vi "_Set Title.vi"(8 "error in (no error)":errorcluster, 9 "Title":string, 10 "Index":i32, 11 "Item_Refnums_Array":T1[](array[typedef])) -> (0 "error out":errorcluster, 3 "Item_Refnums_Array Out":T1[](array[typedef]))   [LabVIEW 2013, in "UI Panels.lvlib" / "Panels_XControl.xctl"]
uses:
  Panels_XControl.xctl
  Controls/References/Panel_Refnums.ctl
  Controls/Panel_Command_Enum.ctl
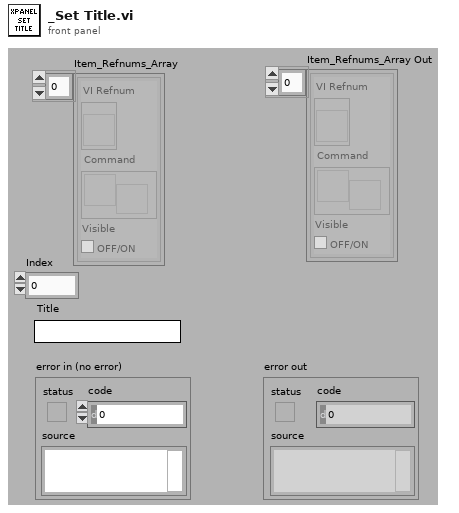
[diagram p1: front panel]
types:
  T1 = typedef "UI Panels.lvlib/Panels_XControl.xctl/Panel_Refnums.ctl" = cluster{"VI Refnum":refnum<vi>, "Command":refnum<user-event>, "Visible":bool}
  T2 = typedef "UI Panels.lvlib/Panels_XControl.xctl/Panel_Command_Enum.ctl" = enum16{"Idle", "Remove & Stop", "Add Item", "Delete Item", "Delete All", "Insert into Subpanel", "Register Menu Events", "Update Value", "Remove from Subpanel", "Set Title", "Set Menu Items", "Insert SubPanel", "Set Splitter Position", "Set Splitter Properties", "Add Menu Items"}
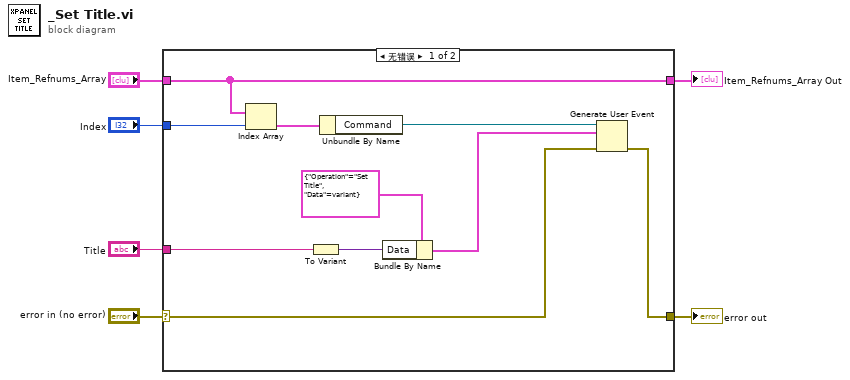
[diagram p0: block diagram]
diagram:
  n1 = case shown="无错误" "error in (no error)" {
    selector: "error in (no error)" -> [w7 w17]
    tunnel: "Index" -> [w15 _]
    tunnel: "Item_Refnums_Array" -> [w11 w18]
    tunnel: "Title" -> [w13 _]
    tunnel: [w9 w17] -> w3
    tunnel: [w11 w18] -> w2
    frame No Error {
      n2 = Index Array(array=w11, index=w15) -> (element=w14:T1)
      n3 = To Variant(anything=w13) -> (Variant=w12:variant)
      n4 = Unbundle By Name(w14) -> ("Command"=w8:refnum<user-event>)
      n5 = Bundle By Name(cluster=cluster{"Operation":T2, "Data":variant} {"Operation"=enum."Set Title", "Data"=variant} ("Item_Command"), "Data"=w12) -> (w10:cluster{"Operation":T2, "Data":variant})
      n6 = Generate User Event(user event=w8, event data cluster=w10, error in=w7) -> (error out=w9:errorcluster)  [unwired: 1 in, 1 out]
    }
    frame Error {
    }
  }
  "Item_Refnums_Array Out" <- w2
  "error out" <- w3
